vi "Pack FXP18.vi"(0 "data in":fxp<+/-,18,1>[](array[numeric])=[0.0, 0.0, 0.0, 0.0, 0.0, 0.0, 0.0, 0.0], 2 "reset":bool, 5 "input valid":bool, 9 "enable bit packing? (T)":bool=TRUE, 12 "ready for output (T)":bool=TRUE) -> (4 "data out":i16[](array[numeric]), 6 "output valid":bool, 14 "ready for input":bool)   [LabVIEW 2018, in "GettingStarted_5774_FPGA.lvlib"]
doc: "Packs an array of FXP<+-,18,1> to an array of I16s.\n\nIf the <B>enable bit packing?</B> input is false, then the FXP<+-,18,1> input elements are converted to FXP<+-,16,1> elements, then the 16-bit elements are returned on the output as an array of I16s.\n\nIf the <B>enable bit packing?</B> input is true, then the FXP<+-,18,1> input elements are converted to FXP<+-,12,1> elements, then the 12-bit elements are packed into 16-bit elements and returned on the output as an array of I16s."
uses:
  <instrlib>/_niInstr/Data Formatting/v1/FPGA/Private/Convert/FXP(+-,12,1) array to Boolean Array.vi
  <instrlib>/_niInstr/Data Formatting/v1/FPGA/Private/Pack/Pack Impl.vi
  <instrlib>/_niInstr/Data Formatting/v1/FPGA/Private/Convert/Boolean Array to U16 Array.vi
  GettingStarted_5774_FPGA.lvlib
  <instrlib>/_niInstr/Data Formatting/v1/FPGA/niInstr Data Formatting v1 FPGA.lvlib
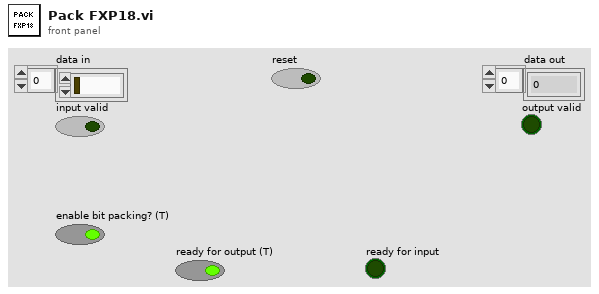
[diagram p1: front panel]
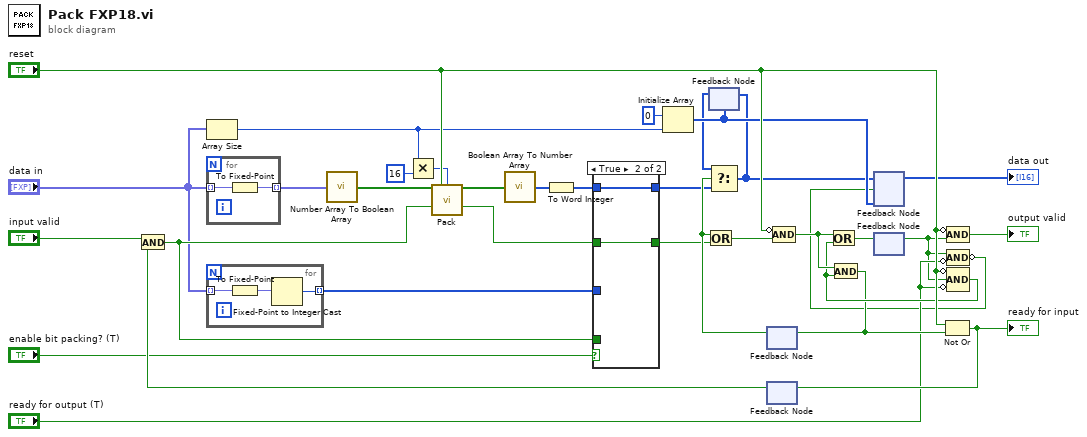
[diagram p0: block diagram]
diagram:
  n1 = Array Size(array="data in") -> (size(s)=w4:i32)
  n2 = for {
    tunnel: "data in" -> [w36] mode=indexing
    tunnel: [w35] -> w3 mode=indexing
    n3 = To Fixed-Point(number=w36) -> (fixed-point=w35:fxp<+/-,12,1>)  [unwired: 1 in]
  }
  n4 = for {
    tunnel: "data in" -> [w39] mode=indexing
    tunnel: [w37] -> w1 mode=indexing
    n5 = To Fixed-Point(number=w39) -> (fixed-point=w38:fxp<+/-,16,1>)  [unwired: 1 in]
    n6 = Fixed-Point to Integer Cast(1:w38) -> (0:w37:i16)
  }
  n7 = call-poly <instrlib>:"Number Array To Boolean Array.vi"("data in"=w3) -> ("data out"=w12:bool[])  [unwired: 14 in]
  n8 = Multiply(x=w4, y=16 ("x")) -> (x*y=w5:i32)
  n9 = Initialize Array(i16 0 ("element"), w4) -> (w33:i16[])
  n10 = feedback #1(w33) -> (w19:i16[])
  n11 = feedback #2() -> (w30:bool)  [unwired: 1 in]
  n12 = feedback #3() -> (w28:bool)  [unwired: 1 in]
  n13 = And(x="input valid", y=w28) -> (x .and. y?=w15:bool)
  n14 = call-poly <instrlib>:"Pack.vi"("data in"=w12, "reset"="reset", "number of output data elements"=w5, "input valid"=w15) -> ("data out"=w11:bool[], "output valid"=w18:bool)  [unwired: 8 in, 2 out]
  n15 = call-poly <instrlib>:"Boolean Array To Number Array.vi"("data in"=w11) -> ("data out"=w10:u16[])  [unwired: 14 in]
  n16 = To Word Integer(number=w10) -> (16bit integer=w9:i16[])
  n17 = case shown="True" "enable bit packing? (T)" {
    tunnel: w9 -> [_ w43]
    tunnel: w1 -> [w41 _]
    tunnel: w15 -> [w40 _]
    tunnel: w18 -> [_ w42]
    tunnel: [w41 w43] -> w17
    tunnel: [w40 w42] -> w14
    frame False {
    }
    frame True {
    }
  }
  n18 = Or(x=w30, y=w14) -> (x .or. y?=w27:bool)
  n19 = Select(t=w19, s=w30, f=w17) -> (s? t:f=w8:i16[])
  n20 = feedback-in #1(w8) -> ()
  n21 = Compound Arithmetic op=AND(invert "reset", w27) -> (w26:bool)
  n22 = feedback #4(w33) -> (→"data out":i16[])
  n23 = feedback #5() -> (w22:bool)  [unwired: 1 in]
  n24 = Compound Arithmetic op=AND(invert "reset", w22) -> (→"output valid":bool)
  n25 = Compound Arithmetic op=AND(w22, invert "ready for output (T)") -> (invert w21:bool)
  n26 = feedback-in #4(w8, w21) -> ()
  n27 = Compound Arithmetic op=AND(invert "reset", w22, invert "ready for output (T)") -> (w25:bool)
  n28 = Or(x=w26, y=w25) -> (x .or. y?=w32:bool)
  n29 = And(x=w26, y=w25) -> (x .and. y?=w24:bool)
  n30 = feedback-in #2(w24) -> ()
  n31 = feedback-in #5(w32) -> ()
  n32 = Not Or(1:w24, 2:"reset") -> (0:w29:bool)
  "ready for input" <- w29
  n33 = feedback-in #3(w29) -> ()
